vi "guarda_archivo.vi"(1 "M or S":bool=TRUE, 2 "Eeprom D-cod":T2 {"Analogicas 32"."?" items=["1", "2", "4", "8", "16", "32", "64", "128", "256"]; "Analogicas 32"."?" items=["Lineal"=15, "Cuadrática"=14]; "Analogicas 32"."unsigned byte array[0]" items=["1"=3, "2"=7, "4"=11, "10"=2, "20"=6, "40"=10, "100"=1, "200"=5, "400"=9, "1000"=0, "2000"=4, "4000"=8]; "Analogicas 16"."?" items=["1", "2", "4", "8", "16", "32", "64", "128", "256"]; "Analogicas 16"."?" items=["Lineal"=15, "Cuadrática"=14]; "Analogicas 16"."unsigned byte array[0]" items=["1"=3, "2"=7, "4"=11, "10"=2, "20"=6, "40"=10, "100"=1, "200"=5, "400"=9, "1000"=0, "2000"=4, "4000"=8]}, 3 "Mediciones 2":T1, 4 "file path nvo":path=path "C:/Documents and Settings/All Users/Documentos/LabVIEW Data/Soft Telemedicion/Beta 2.2/Equipo1/09-06-18.xls") -> (0 "error out":errorcluster)   [LabVIEW 2010]
uses:
  <vilib>/Utility/file.llb/Write To Spreadsheet File (string).vi
panel:
  out "error out 2":errorcluster
  out "grabó ok":bool
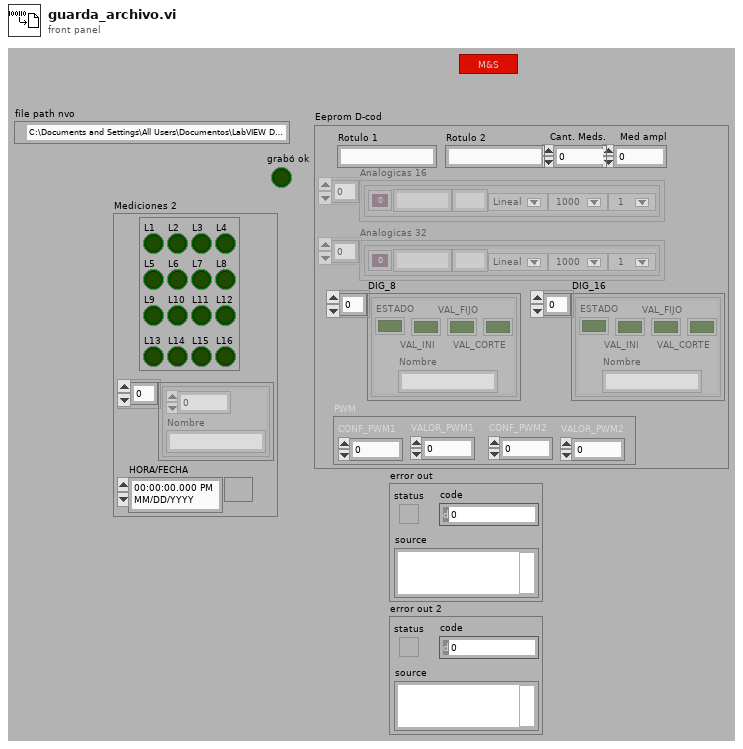
[diagram p1: front panel]
types:
  T1 = cluster{cluster{"L1":bool, "L2":bool, "L3":bool, "L4":bool, "L5":bool, "L6":bool, "L7":bool, "L8":bool, "L9":bool, "L10":bool, "L11":bool, "L12":bool, "L13":bool, "L14":bool, "L15":bool, "L16":bool}, cluster{dbl, "Nombre":string}[], "HORA/FECHA":timestamp}
  T2 = cluster{"Rotulo 1":string, "Rotulo 2":string, "Cant. Meds.":u8, "Med ampl":u8, "Analogicas 16":cluster{i32, "mapaeeprom":string, "mapaeeprom":string, u8, "unsigned byte array[0]":u8, u8}[], "Analogicas 32":cluster{i32, "mapaeeprom":string, "mapaeeprom":string, u8, "unsigned byte array[0]":u8, u8}[], "DIG_8":cluster{"ESTADO":bool, "VAL_INI":bool, "VAL_FIJO":bool, "VAL_CORTE":bool, "Nombre":string}[], "DIG_16":cluster{"ESTADO":bool, "VAL_INI":bool, "VAL_FIJO":bool, "VAL_CORTE":bool, "Nombre":string}[], "PWM":cluster{"CONF_PWM1":u8, "VALOR_PWM1":u8, "CONF_PWM2":u8, "VALOR_PWM2":u8}}
  T3 = enum16{"open", "replace", "create", "open or create", "replace or create", "replace or create with confirmation"}
  T4 = cluster{i32, "mapaeeprom":string, "mapaeeprom":string, u8, "unsigned byte array[0]":u8, u8}[]
  T5 = cluster{"[0]":cluster{i32, "mapaeeprom":string, "mapaeeprom":string, u8, "unsigned byte array[0]":u8, u8}}
  T6 = cluster{i32, "mapaeeprom":string, "mapaeeprom":string, u8, "unsigned byte array[0]":u8, u8}
  T7 = cluster{"L1":bool, "L2":bool, "L3":bool, "L4":bool, "L5":bool, "L6":bool, "L7":bool, "L8":bool, "L9":bool, "L10":bool, "L11":bool, "L12":bool, "L13":bool, "L14":bool, "L15":bool, "L16":bool}
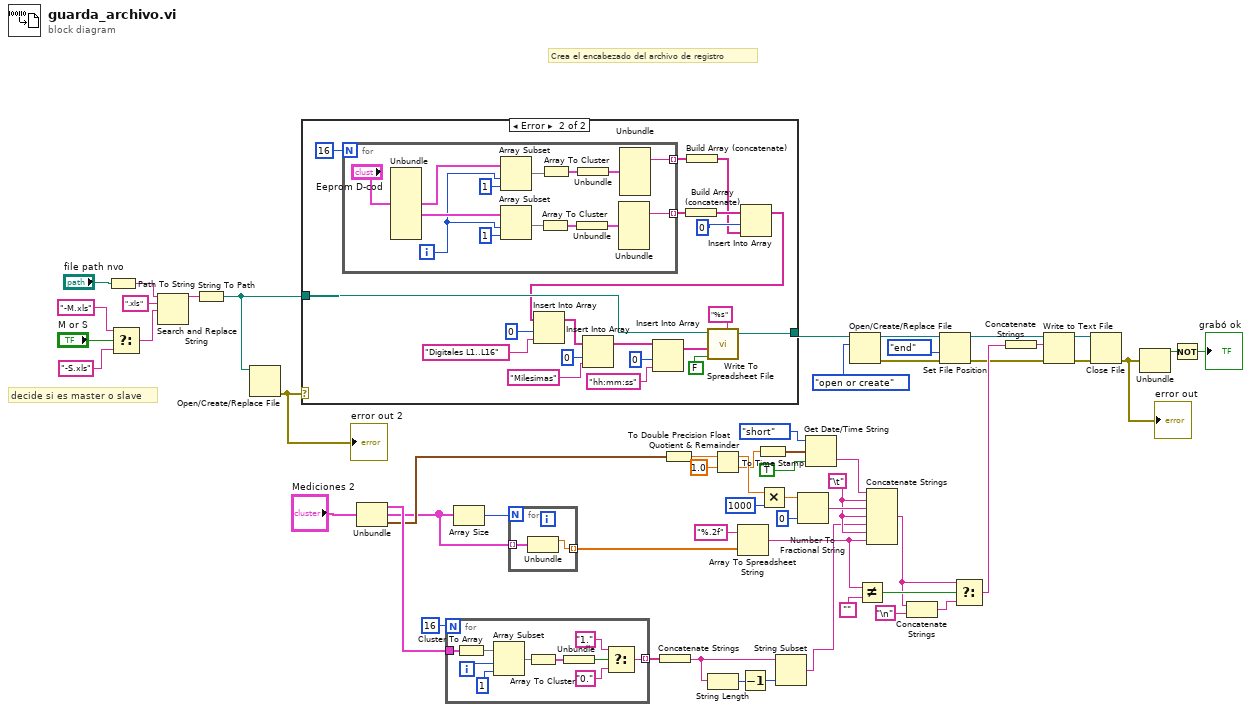
[diagram p0: block diagram]
diagram:
  w33 = "\t"
  # "decide si es master o slave"
  # "Crea el encabezado del archivo de registro"
  n1 = Path To String(path="file path nvo") -> (string=w7:string)
  n2 = Select(t="-M.xls" ("search string"), s="M or S", f="-S.xls" ("search string")) -> (s? t:f=w2:string)
  n3 = Search and Replace String(input string=w7, search string=".xls", replace string=w2) -> (result string=w1:string)  [unwired: 5 in, 3 out]
  n4 = String To Path(string=w1) -> (path=w8:path)
  n5 = Open/Create/Replace File(file path (use dialog)=w8) -> (error out=w17:errorcluster)  [unwired: 2 in, 5 out]
  "error out 2" <- w17
  n6 = case shown="Error" w17 {
    tunnel: [w57 w67] -> w16
    tunnel: w8 -> [w57 w65]
    frame No Error {
    }
    frame Error {
      n7 = for {
        N: 16 -> [_]
        tunnel: [w80] -> w62 mode=indexing
        tunnel: [w79] -> w63 mode=indexing
        i -> [w78]
        n8 = Unbundle("Eeprom D-cod") -> ("Analogicas 16"=w90:T4, "Analogicas 32"=w84:T4)  [unwired: 7 out]
        n9 = Array Subset(array=w90, index=w78, length=1) -> (w88:T4)
        n10 = Array Subset(array=w84, index=w78, length=1) -> (w81:T4)
        n11 = Array To Cluster(array=w81) -> (cluster=w82:T5)
        n12 = Array To Cluster(array=w88) -> (cluster=w87:T5)
        n13 = Unbundle(w82) -> ("[0]"=w83:T6)
        n14 = Unbundle(w87) -> ("[0]"=w86:T6)
        n15 = Unbundle(w83) -> ("mapaeeprom"=w80:string)  [unwired: 5 out]
        n16 = Unbundle(w86) -> ("mapaeeprom"=w79:string)  [unwired: 5 out]
      }
      n17 = Build Array (concatenate)(w62) -> (w59:string[])
      n18 = Build Array (concatenate)(w63) -> (w58:string[])
      n19 = Insert Into Array(array=w59, index=0, new element=w58) -> (w60:string[])
      n20 = Insert Into Array(array=w60, index=0, new element="Digitales L1..L16" ("new element/subarray")) -> (w75:string[])
      n21 = Insert Into Array(array=w75, index=0, new element="Milesimas" ("new element/subarray")) -> (w73:string[])
      n22 = Insert Into Array(array=w73, index=0, new element="hh:mm:ss" ("new element/subarray")) -> (w72:string[])
      n23 = call-poly <vilib>:"Write To Spreadsheet File.vi"("format (%s)"="%s", "append to file? (new file:F)"=FALSE, "1D data"=w72, "file path (dialog if empty)"=w65) -> ("new file path (Not A Path if cancelled)"=w67:path)  [unwired: 2 in, 2 out]
    }
  }
  n24 = Unbundle("Mediciones 2") -> (w23:T7, w11:cluster{dbl, "Nombre":string}[], "HORA/FECHA"=w22:timestamp)
  n25 = for {
    N: 16 -> [_]
    tunnel: [w97] -> w31 mode=indexing
    tunnel: w23 -> [w94]
    i -> [w98]
    n26 = Cluster To Array(cluster=w94) -> (array=w93:bool[])
    n27 = Array Subset(array=w93, index=w98, length=1) -> (w101:bool[])
    n28 = Array To Cluster(array=w101) -> (cluster=w100:cluster{"[0]":bool})
    n29 = Unbundle(w100) -> ("[0]"=w92:bool)
    n30 = Select(t="1.", s=w92, f="0.") -> (s? t:f=w97:string)
  }
  n31 = Array Size(array=w11) -> (size(s)=w12:i32)
  n32 = for {
    N: w12 -> [_]
    tunnel: w11 -> [w103] mode=indexing
    tunnel: [w102] -> w10 mode=indexing
    n33 = Unbundle(w103) -> (w102:dbl)  [unwired: 1 out]
  }
  n34 = Concatenate Strings(w31) -> (w19:string)
  n35 = To Double Precision Float(number=w22) -> (double precision float=w30:dbl)
  n36 = String Length(string=w19) -> (length=w21:i32)
  n37 = Quotient & Remainder(x=w30, y=1.0) -> (x-y*floor(x/y)=w39:dbl, floor(x/y)=w34:dbl)
  n38 = Array To Spreadsheet String(array=w10, 3:"%.2f" ("format string")) -> (spreadsheet string=w25:string)  [unwired: 1 out]
  n39 = Decrement(x=w21) -> (x-1=w20:i32)
  n40 = To Time Stamp(1:w34) -> (0:w37:timestamp)
  n41 = Multiply(x=w39, y=1000 ("index")) -> (x*y=w43:dbl)
  n42 = String Subset(string=w19, length (rest)=w20) -> (substring=w18:string)  [unwired: 1 out]
  n43 = Number To Fractional String(number=w43, precision (6)=i16 0) -> (F-format string=w42:string)  [unwired: 2 out]
  n44 = Get Date/Time String(date format (0)=enum16{"short", "long", "abbreviated"}."short", seconds (now)=w37, want seconds? (F)=TRUE) -> (time string=w41:string)  [unwired: 1 out]
  n45 = Open/Create/Replace File(file path (use dialog)=w16, operation (0:open)=T3."open or create") -> (refnum out=w55:refnum<file>, error out=w15:errorcluster)  [unwired: 1 in, 4 out]
  n46 = Not Equal?(x=w25, y="") -> (x != y?=w29:bool)
  n47 = Concatenate Strings(w41, w33, w42, w33, w18, w33, w25) -> (w28:string)
  n48 = Concatenate Strings(w28, "\n") -> (w27:string)
  n49 = Set File Position(refnum=w55, from (0:start)=enum16{"start", "end", "current"}."end", error in=w15) -> (refnum out=w51:refnum<file>, error out=w14:errorcluster)  [unwired: 1 out]
  n50 = Select(t=w28, s=w29, f=w27) -> (s? t:f=w50:string)
  n51 = Concatenate Strings(w50) -> (w49:string)
  n52 = Write to Text File(file (use dialog)=w51, text=w49, error in=w14) -> (refnum out=w53:refnum<file>, error out=w52:errorcluster)  [unwired: 2 out]
  n53 = Close File(refnum=w53, error in=w52) -> (error out=w48:errorcluster)  [unwired: 1 out]
  "error out" <- w48
  n54 = Unbundle(w48) -> ("status"=w47:bool)  [unwired: 2 out]
  n55 = Not(x=w47) -> (.not. x?=→"grabó ok":bool)
